vi "CalibrationSavePrompt.vi"(0 "Root Path":path) -> (1 "selected path":path, 2 "cancel?":bool)   [LabVIEW 2024]
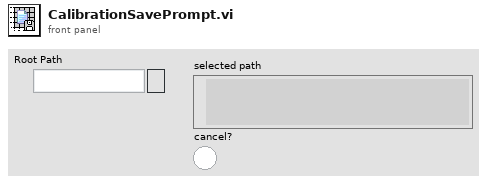
[diagram p1: front panel]
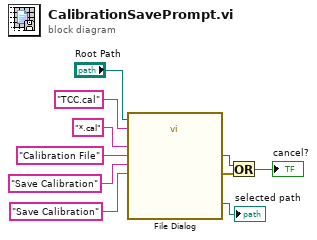
[diagram p0: block diagram]
diagram:
  n1 = call "File Dialog"("start path"="Root Path", "prompt"="Save Calibration", "button label"="Save Calibration", "default name"="TCC.cal", "pattern (all files)"="*.cal", "pattern label"="Calibration File") -> ("selected path"=→"selected path":path, "cancelled"=w9:bool, "error out"=w10:errorcluster)  [unwired: 6 in, 1 out]
  n2 = Or(x=w9, y=w10) -> (x .or. y?=→"cancel?":bool)
